vi "Navigate - Refactored.vi"(1 "Pathfinding Settings":T1={"Movement Settings"={"Arrival Tolerance (m)"=0.01, "Closeness Threshold (m)"=0.5, "Pit Obstacle Radius (m)"=0.5, "Pit Locations"=[]}, "Dead Zone"=0.75, "Max Moves"=3.0, "Move Segment Length (m)"=0.02, "Path Cost Weights"={"Length Weight"=1.0, "Angle Weight"=0.0, "Angle Error Weight"=1000.0, "Angle Error Threshold"=0.314, "Per Move Penalty"=0.05, "Closeness Weight"=100.0, "Too Short Penalty"=100.0, "Too Short Threshold"=1.5}, "Desperation - Reduction Per Attempt (Ratio)"=0.9, "Desperation - Max Attempts"=1, "Log All Move Points"=FALSE, "Intermediate Position Grids"=[{"x1"=0.0, "x2"=1.75, "resolution"=0.15}, {"x1"=1.75, "x2"=7.38, "resolution"=0.4}]}, 2 "Move Type":T5(ring)) -> ()   [LabVIEW 2015, in "Navigation2017.lvlib"]
uses:
  Navigation2017.lvlib
  PathfindingSettings.ctl
  MovementSettings.ctl
  PathCostWeights.ctl
  IntermediatePositionGrids.ctl
  Vector.ctl
  PathOfMoves.ctl
  Move.ctl
  Navigation2017-util.lvlib
panel:
  out "Pathfinding Loop Count":i32
  in  "Reached Next Path Point Threshold Distance (m)":dbl(knob)=0.2054620332336267 scale=0.0..1.0
  in  "Robot Speed":dbl(slide)=1.0 scale=0.0..1.0
  in  "Dead Reckoning Move Distance (m)":dbl(knob)=1.1303212530968743 scale=0.5..4.0
  in  "Turning Radius (m)":dbl(knob)=0.75 scale=0.75..4.0
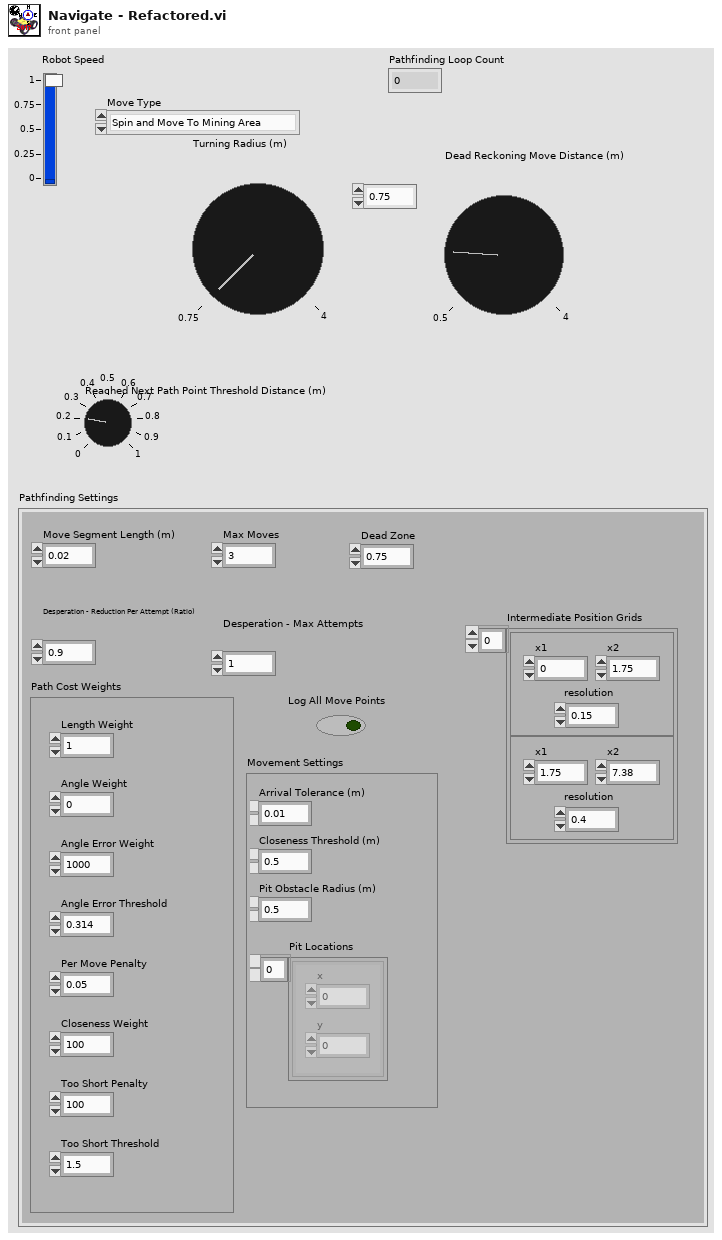
[diagram p1: front panel]
types:
  T1 = typedef "Navigation2017.lvlib/PathfindingSettings.ctl" = cluster{"Movement Settings":T2, "Dead Zone":dbl, "Max Moves":dbl, "Move Segment Length (m)":dbl, "Path Cost Weights":T3, "Desperation - Reduction Per Attempt (Ratio)":dbl, "Desperation - Max Attempts":i16, "Log All Move Points":bool, "Intermediate Position Grids":T4}
  T2 = typedef "Navigation2017.lvlib/MovementSettings.ctl" = cluster{"Arrival Tolerance (m)":dbl, "Closeness Threshold (m)":dbl, "Pit Obstacle Radius (m)":dbl, "Pit Locations":cluster{"x":dbl, "y":dbl}[]}
  T3 = typedef "Navigation2017.lvlib/PathCostWeights.ctl" = cluster{"Length Weight":dbl, "Angle Weight":dbl, "Angle Error Weight":dbl, "Angle Error Threshold":dbl, "Per Move Penalty":dbl, "Closeness Weight":dbl, "Too Short Penalty":dbl, "Too Short Threshold":dbl}
  T4 = typedef "Navigation2017.lvlib/IntermediatePositionGrids.ctl" = cluster{"x1":dbl, "x2":dbl, "resolution":dbl}[]
  T5 = enum16{"Spin and Move To Mining Area", "Move To Collector Trough", "Move To Mining Area"}
  T6 = typedef "Navigation2017.lvlib/Vector.ctl" = cluster{"x":dbl, "y":dbl, "angle":dbl}
  T7 = typedef "Navigation2017.lvlib/PathOfMoves.ctl" = cluster{"Dest Angle Error":dbl, "Dest Angle Considered":bool, "Moves":T8[]}
  T8 = typedef "Navigation2017.lvlib/Move.ctl" = cluster{"Did Reach Dest":bool, "Did Collide":bool, "Sum of Angle Changes (rad)":dbl, "Move Length (m)":dbl, "Closeness Sum":dbl, "Positions Along Move":T6[], "Moved Fwd":bool}
  T9 = typedef "LocalizationStatus.ctl" = cluster{"x":dbl, "y":dbl, "angle":dbl, "valid":bool, "lastUpdatedTime":dbl}
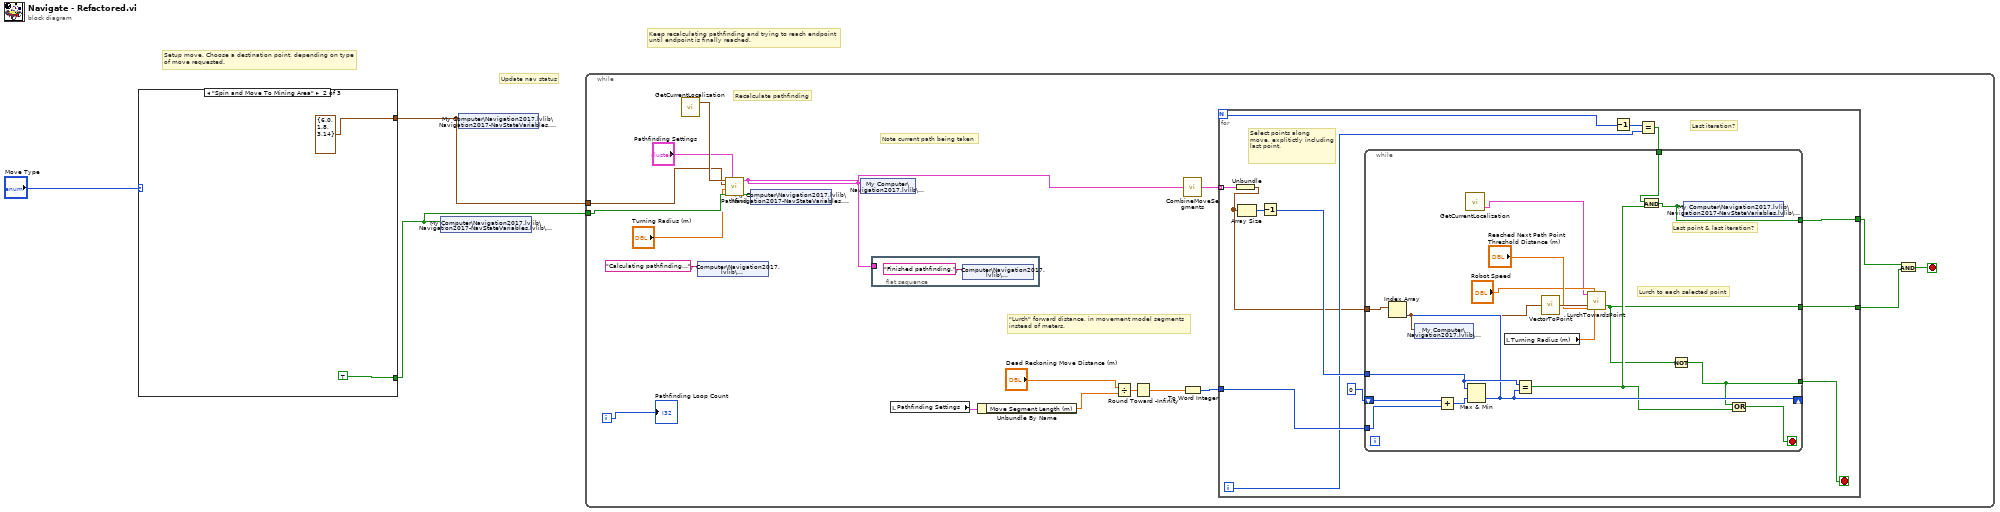
[diagram p0: block diagram]
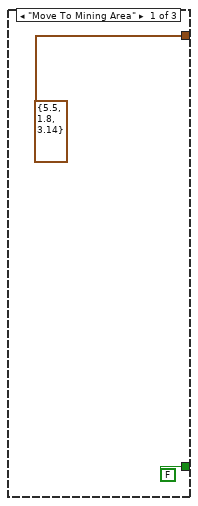
[diagram p2: hidden frame]
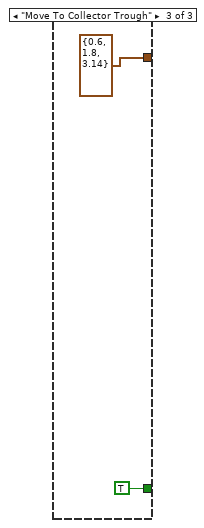
[diagram p3: hidden frame]
diagram:
  # "Keep recalculating pathfinding and trying to reach endpoint\nuntil endpoint is finally reached."
  # "Update nav status"
  # "Setup move. Choose a destination point, depending on type\nof move requested."
  n1 = case shown="\"Spin and Move To Mining Area\"" "Move Type" {
    tunnel: [T6 {"x"=5.5, "y"=1.8, "angle"=3.14} ("Vector") T6 {"x"=6.0, "y"=1.8, "angle"=3.14} ("Vector") T6 {"x"=0.6, "y"=1.8, "angle"=3.14} ("Vector")] -> w2
    tunnel: [FALSE TRUE TRUE] -> w1
    frame "Move To Mining Area" {
    }
    frame "Spin and Move To Mining Area" {
    }
    frame "Move To Collector Trough" {
    }
  }
  n2 = shared-variable "My Computer\\Navigation2017.lvlib\\Navigation2017-NavStateVariables.lvlib\\SpecifyingEndAngle"(w1) -> ()  [unwired: 1 in, 1 out]
  n3 = shared-variable "My Computer\\Navigation2017.lvlib\\Navigation2017-NavStateVariables.lvlib\\DestinationPoint"(w2) -> ()  [unwired: 1 in, 1 out]
  n4 = while {
    tunnel: w2 -> [w26]
    tunnel: w1 -> [w25]
    i -> [w28]
    stop <- w11 stop-if-true
    # "\"Lurch\" forward distance, in movement model segments\ninstead of meters."
    # "Note current path being taken"
    # "Recalculate pathfinding"
    n5 = call "GetCurrentLocalization.vi"() -> ("Current Localization Vector"=w27:T6)  [unwired: 1 out]
    n6 = shared-variable "My Computer\\Navigation2017.lvlib\\Navigation2017-NavStateVariables.lvlib\\CurrNavStage"("Calculating pathfinding..." ("CurrNavStage")) -> ()  [unwired: 1 in, 1 out]
    n7 = call "Pathfind.vi"("Pathfinding Settings"="Pathfinding Settings", "Specified End Angle"=w25, "Turn Radius (m)"="Turning Radius (m)", "Destination"=w26, "Start Vector"=w27) -> ("Desperation Used"=w22:bool, "Best Path"=w16:T7)  [unwired: 3 out]
    n8 = shared-variable "My Computer\\Navigation2017.lvlib\\Navigation2017-NavStateVariables.lvlib\\UsedDesperation"(w22) -> ()  [unwired: 1 in, 1 out]
    n9 = shared-variable "My Computer\\Navigation2017.lvlib\\Navigation2017-NavStateVariables.lvlib\\CurrPath"(w16) -> ()  [unwired: 1 in, 1 out]
    n10 = flat-sequence {
      tunnel: w16 -> [_]
      frame #0 {
        n11 = shared-variable "My Computer\\Navigation2017.lvlib\\Navigation2017-NavStateVariables.lvlib\\CurrNavStage"("Finished pathfinding." ("CurrNavStage")) -> ()  [unwired: 1 in, 1 out]
      }
    }
    n12 = local read "Pathfinding Settings"() -> (w17:T1)
    n13 = Unbundle By Name(w17) -> ("Move Segment Length (m)"=w18:dbl)
    n14 = Divide(x="Dead Reckoning Move Distance (m)", y=w18) -> (x/y=w20:dbl)
    n15 = Round Toward -Infinity(1:w20) -> (0:w14:dbl)
    n16 = call "CombineMoveSegments.vi"("Path"=w16) -> ("Combined Moves & Positions"=w10:cluster{T6[]}[])
    n17 = To Word Integer(number=w14) -> (16bit integer=w15:i16)
    n18 = for {
      N -> [w36]
      tunnel: w15 -> [w41]
      tunnel: [w32] -> w13
      tunnel: [w31] -> w12
      tunnel: w10 -> [w30] mode=indexing
      i -> [w34]
      stop <- w37 stop-if-true
      # "Last iteration?"
      # "Select points along\nmove, explitictly including last point."
      n19 = Unbundle(w30) -> (w29:T6[])
      n20 = Array Size(array=w29) -> (size(s)=w39:i32)
      n21 = Decrement(x=w39) -> (x-1=w38:i32)
      n22 = Decrement(x=w36) -> (x-1=w35:i32)
      n23 = Equal?(x=w35, y=w34) -> (x = y?=w33:bool)
      n24 = while {
        shift-right: [w54] -> _
        shift-left: i16 0 -> [w58]
        tunnel: w41 -> [w59]
        tunnel: w38 -> [w56]
        tunnel: w29 -> [w53]
        tunnel: [w48] -> w37
        tunnel: w33 -> [w46]
        tunnel: [w45] -> w32
        tunnel: [w44] -> w31
        stop <- w49 stop-if-true
        # "Last point & last iteration?"
        # "Lurch to each selected point"
        n25 = Add(x=w58, y=w59) -> (x+y=w57:i32)
        n26 = call "GetCurrentLocalization.vi"() -> ("Current Localization Status"=w42:T9)  [unwired: 1 out]
        n27 = Max & Min(x=w56, y=w57) -> (min(x,y)=w54:i32)  [unwired: 1 out]
        n28 = Index Array(array=w53, index=w54) -> (element=w43:T6)
        n29 = shared-variable "My Computer\\Navigation2017.lvlib\\Navigation2017-NavStateVariables.lvlib\\NextPoint"(w43) -> ()  [unwired: 1 in, 1 out]
        n30 = local read "Turning Radius (m)"() -> (w50:dbl)
        n31 = Equal?(x=w56, y=w54) -> (x = y?=w47:bool)
        n32 = call "VectorToPoint.vi"("Vector"=w43) -> ("Point"=w55:cluster{"x":dbl, "y":dbl})
        n33 = call "LurchTowardsPoint.vi"("Turning Radius (m)"=w50, "Robot Speed"="Robot Speed", "Reached Next Path Point Threshold Distance (m)"="Reached Next Path Point Threshold Distance (m)", "Dest. Point"=w55, "Curr Localization Status"=w42) -> ("Within Tolerance of Dest"=w44:bool)  [unwired: 1 in, 1 out]
        n34 = And(x=w46, y=w47) -> (x .and. y?=w45:bool)
        n35 = Not(x=w44) -> (.not. x?=w48:bool)
        n36 = shared-variable "My Computer\\Navigation2017.lvlib\\Navigation2017-NavStateVariables.lvlib\\NextPointIsDestination"(w45) -> ()  [unwired: 1 in, 1 out]
        n37 = Or(x=w48, y=w47) -> (x .or. y?=w49:bool)
      }
    }
    n38 = And(x=w13, y=w12) -> (x .and. y?=w11:bool)
    "Pathfinding Loop Count" <- w28
  }
